vi "PNACreateMeas.vi"(5 "Meas in":T1={"S11"=TRUE, "S12"=TRUE, "S21"=TRUE, "S22"=TRUE}) -> (0 "Disp traces":i32[](array[numeric]), 1 "Disp windows":i32[](array[numeric]), 2 "Disp format":i32[](array[ring]) items=["Magnitude Logarithmic", "Magnitude Linear", "Phase", "Smith Chart", "Polar", "Real", "Imaginary", "SWR", "Group Delay", "Unwrapped phase", "Smith Admittance"], 3 "Meas types":i32[](array[ring]) items=["S11", "S12", "S21", "S22", "A", "B", "R1", "R2", "A/B", "B/A"], 4 "Meas names":string[](array[string])=["MEAS0", "MEAS1", "MEAS2", "MEAS3"])   [LabVIEW 2017]
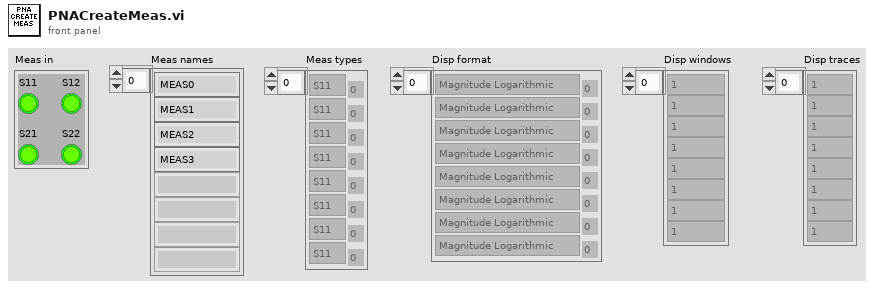
[diagram p1: front panel]
types:
  T1 = cluster{"S11":bool, "S12":bool, "S21":bool, "S22":bool}
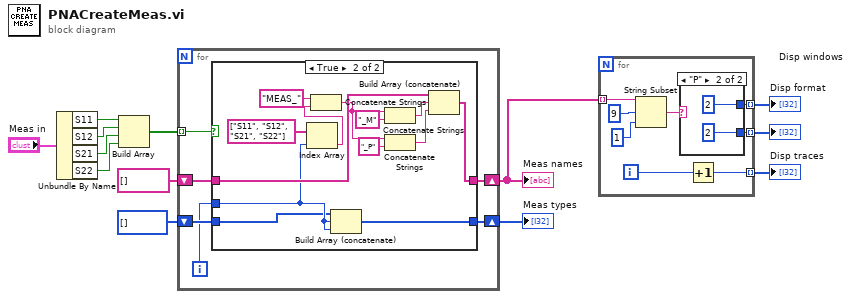
[diagram p0: block diagram]
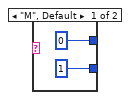
[diagram p2: hidden frame]
diagram:
  n1 = Unbundle By Name("Meas in") -> ("S11"=w12:bool, "S12"=w11:bool, "S21"=w10:bool, "S22"=w9:bool)
  n2 = Build Array(w12, w11, w10, w9) -> (w8:bool[])
  n3 = for {
    tunnel: w8 -> [w19] mode=indexing
    shift-right: [w17] -> w4
    shift-left: string[] [] ("appended array") -> [w18]
    shift-right: [w15] -> w5
    shift-left: i32[] [] ("appended array") -> [w16]
    i -> [w14]
    n4 = case shown="True" w19 {
      tunnel: w18 -> [w21 w33]
      tunnel: [w21 w32] -> w17
      tunnel: w14 -> [_ w23]
      tunnel: w16 -> [w20 w22]
      tunnel: [w20 w31] -> w15
      frame False {
      }
      frame True {
        n5 = Index Array(array=string[] ["S11", "S12", "S21", "S22"] ("appended array"), index=w23) -> (element=w29:string)
        n6 = Concatenate Strings("MEAS_", w29) -> (w28:string)
        n7 = Build Array (concatenate)(w22, w23, w23) -> (w31:i32[])
        n8 = Concatenate Strings(w28, "_M" ("string")) -> (w25:string)
        n9 = Concatenate Strings(w28, "_P" ("string")) -> (w24:string)
        n10 = Build Array (concatenate)(w33, w25, w24) -> (w32:string[])
      }
    }
  }
  "Meas names" <- w4
  "Meas types" <- w5
  n11 = for {
    tunnel: w4 -> [w40] mode=indexing
    tunnel: [w41] -> w3 mode=indexing
    tunnel: [w37] -> w2 mode=indexing
    tunnel: [w36] -> w1 mode=indexing
    i -> [w42]
    n12 = String Subset(string=w40, offset (0)=9, length (rest)=1 ("length (rest)")) -> (substring=w35:string)
    n13 = case shown="\"P\"" w35 {
      tunnel: [0 2] -> w37
      tunnel: [1 2] -> w36
      frame "M", Default {
      }
      frame "P" {
      }
    }
    n14 = Increment(x=w42) -> (x+1=w41:i32)
  }
  "Disp format" <- w2
  "Disp traces" <- w3
  "Disp windows" <- w1
